vi "Translation_GetX.vi"(11 "In Translation":T1) -> (3 "X":dbl)   [LabVIEW 2019, in "Trajectory_Library.lvlib"]
doc: "Returns the X component of the translation.\n\nParameters\n - IN Translation - This Translation data structure\n\nReturns:\n - X- The x component of the translation."
uses:
  Trajectory_Library.lvlib
  TRANSLATION2D.ctl
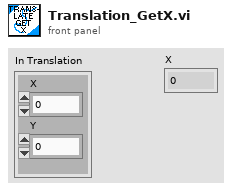
[diagram p1: front panel]
types:
  T1 = typedef "Trajectory_Library.lvlib/TRANSLATION2D.ctl" = cluster{"X":dbl, "Y":dbl}
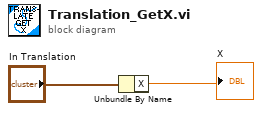
[diagram p0: block diagram]
diagram:
  n1 = Unbundle By Name("In Translation") -> ("X"=→"X":dbl)
